vi "UnitsToCounts.vi"(1 "Unit Value":dbl, 2 "Units":enum16{"mm", "µm"}(ring)) -> (0 "Counts":i32)   [LabVIEW 2023]
doc: "Convert units to counts"
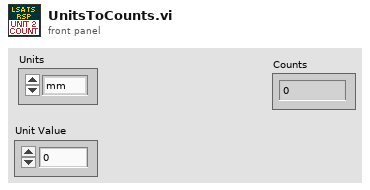
[diagram p1: front panel]
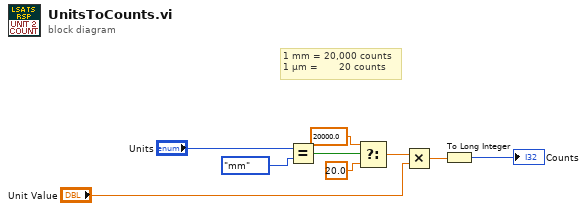
[diagram p0: block diagram]
diagram:
  # "1 mm = 20,000 counts\n1 µm =       20 counts"
  n1 = Equal?(x="Units", y=enum16{"mm", "µm"}."mm" ("Units")) -> (x = y?=w8:bool)
  n2 = Select(t=20000.0, s=w8, f=20.0) -> (s? t:f=w5:dbl)
  n3 = Multiply(x=w5, y="Unit Value") -> (x*y=w9:dbl)
  n4 = To Long Integer(number=w9) -> (32bit integer=→"Counts":i32)
